vi "Info Replace Matrix.vi"(7 "key description to replace":string, 8 "Is Section (False)":bool, 9 "Allow indent (True)":bool=TRUE, 10 "info data to paste":string, 11 "info data in":string) -> (3 "info data out":string)   [LabVIEW 2020]
doc: "Addition to infolib: Replaces matrix section by another string input."
uses:
  <vilib>/Utility/error.llb/whitespace.ctl
  <vilib>/regexp/Match Regular Expression.xnode
panel:
  out "submatch 1":string
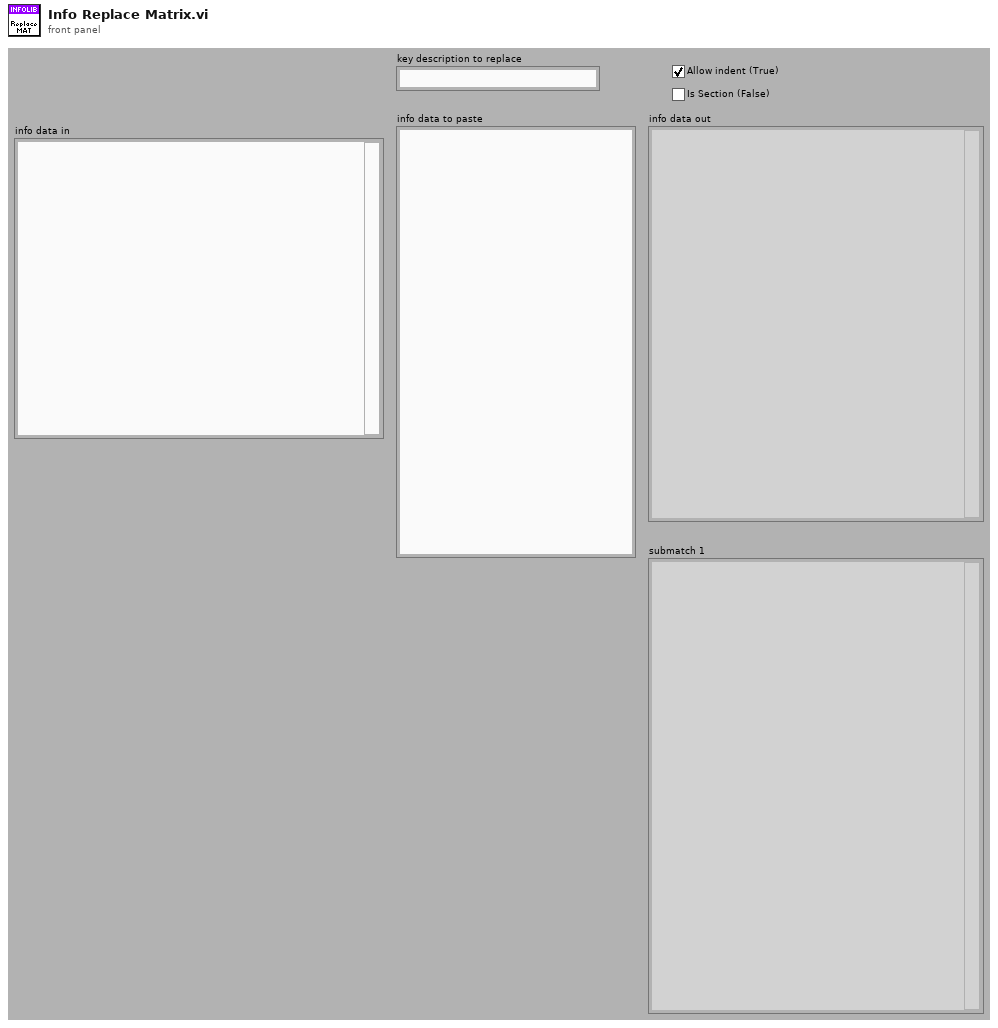
[diagram p1: front panel]
types:
  T1 = typedef "whitespace.ctl" = u16
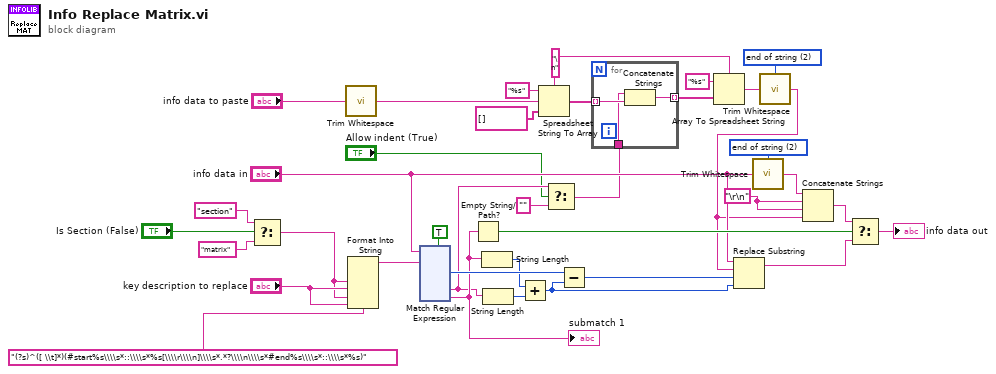
[diagram p0: block diagram]
diagram:
  w1 = T1 2 items=["both", "start of string", "end of string"] ("location (both)")
  w11 = T1 2 items=["both", "start of string", "end of string"] ("location (both)")
  w13 = "\n" ("delimiter (Tab)")
  w2 = "\r\n"
  n1 = Select(t="section" ("f"), s="Is Section (False)", f="matrix") -> (s? t:f=w8:string)
  n2 = call <vilib>:"Trim Whitespace.vi"("string"="info data to paste") -> ("trimmed string"=w22:string)  [unwired: 1 in]
  n3 = Format Into String(format string="(?s)^([ \\t]*)(#start%s\\\\s*::\\\\s*%s[\\\\r\\\\n]\\\\s*.*?\\\\n\\\\s*#end%s\\\\s*::\\\\s*%s)", w8, "key description to replace", w8, "key description to replace") -> (resulting string=w34:string)  [unwired: 2 in, 1 out]
  n4 = xnode "Match Regular Expression"("input string"="info data in", "regular expression"=w34, "multiline? (F)"=TRUE) -> ("offset past match"=w36:i32, "submatch 1"=w17:string, "submatch 2"=w26:string)  [unwired: 3 in, 4 out]
  "submatch 1" <- w26
  n5 = Empty String/Path?(string/path=w26) -> (empty?=w30:bool)
  n6 = String Length(string=w26) -> (length=w25:i32)
  n7 = String Length(string=w17) -> (length=w24:i32)
  n8 = Add(x=w25, y=w24) -> (x+y=w23:i32)
  n9 = Spreadsheet String To Array(delimiter (Tab)=w13, format string="%s", spreadsheet string=w22, array type (2D Dbl)=string[] []) -> (array=w19:string[])
  n10 = Select(t=w17, s="Allow indent (True)", f="") -> (s? t:f=w18:string)
  n11 = Subtract(x=w36, y=w23) -> (x-y=w33:i32)
  n12 = for {
    tunnel: w19 -> [w40] mode=indexing
    tunnel: w18 -> [w39]
    tunnel: [w38] -> w14 mode=indexing
    n13 = Concatenate Strings(w39, w40) -> (w38:string)
  }
  n14 = Array To Spreadsheet String(delimiter (Tab)=w13, array=w14, 3:"%s" ("format string")) -> (spreadsheet string=w5:string)
  n15 = call <vilib>:"Trim Whitespace.vi"("string"="info data in", "location (both)"=w1) -> ("trimmed string"=w3:string)
  n16 = call <vilib>:"Trim Whitespace.vi"("string"=w5, "location (both)"=w11) -> ("trimmed string"=w4:string)
  n17 = Replace Substring(2:w23, 3:w33, 4:w4, 5:"info data in") -> (1:w29:string)  [unwired: 1 out]
  n18 = Concatenate Strings(w3, w2, w2, w4) -> (w28:string)
  n19 = Select(t=w28, s=w30, f=w29) -> (s? t:f=→"info data out":string)
